vi "Read datatype.vi"(8 "error in (no error)":errorcluster, 11 "JSON Datatype in":refnum<class "JSON Null.lvclass">) -> (0 "error out":errorcluster, 2 "datatype":T1, 3 "JSON Datatype out":refnum<class "JSON Null.lvclass">)   [LabVIEW 2015, in "LVJSON.lvlib" / "JSON Null.lvclass"]
doc: "Returns the JSON Type of the given object. This may be used to determine if the value of a control of type JSON Null, JSON Literal or JSON Structured Type is an instance of a more specific type."
uses:
  JSON Null.lvclass
  JSON Types.ctl
  LVJSON.lvlib
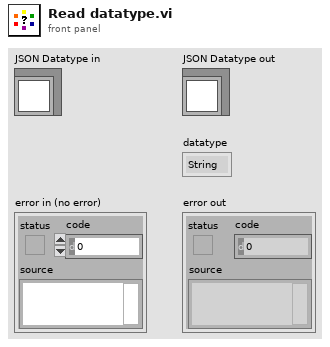
[diagram p1: front panel]
types:
  T1 = typedef "LVJSON.lvlib/JSON Types.ctl" = enum16{"String", "Numeric", "Boolean", "NULL", "Object", "Array"}
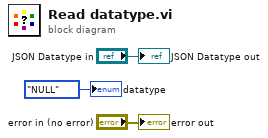
[diagram p0: block diagram]
diagram:
  "error out" <- "error in (no error)"
  "JSON Datatype out" <- "JSON Datatype in"
  "datatype" <- JSON_Types."NULL" ("datatype")
